vi "Get Data.vi"(8 "error in (no error)":errorcluster, 10 "Data Type":string, 11 "Communication in":refnum<class "Communication.lvclass">) -> (0 "error out":errorcluster, 3 "Communication out":refnum<class "Communication.lvclass">)   [LabVIEW 2023, in "Communication.lvclass"]
uses:
  Communication.lvclass
  Data/Data.lvclass
  Controls/User Event Operation.ctl
  Downloads/Sample PC Template/Sample PC Template/Typedefs/Data.ctl
  Communication.lvclass/Communication.ctl
  Downloads/Sample PC Template/Sample PC Template/Sample PC Template.lvlib
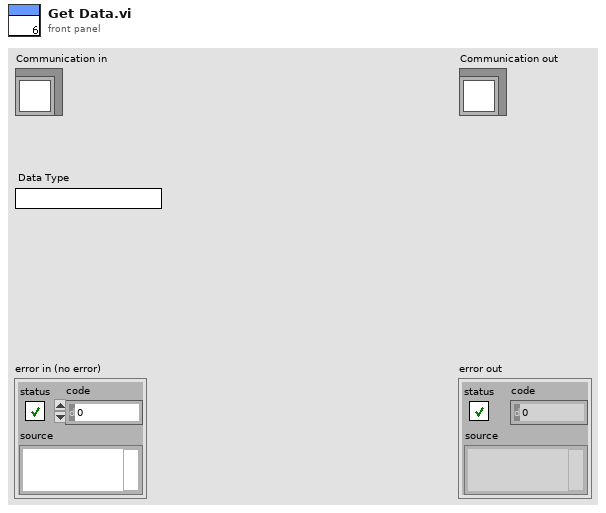
[diagram p1: front panel]
types:
  T1 = typedef "Sample PC Template.lvlib/Data.ctl" = cluster{"State":string, "Data":variant}
  T2 = typedef "User Event Operation.ctl" = enum16{"Obtain", "Generate", "Release"}
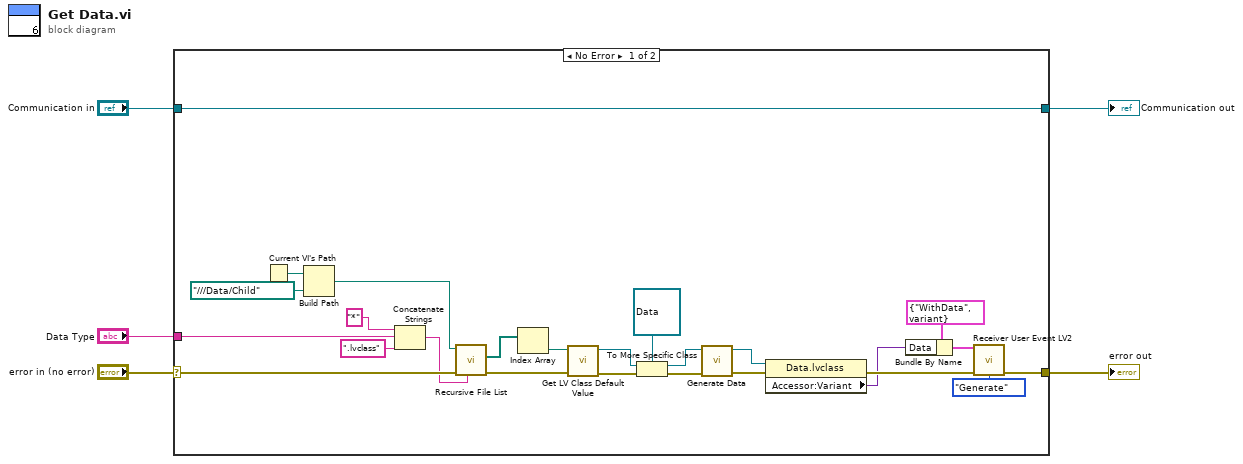
[diagram p0: block diagram]
diagram:
  n1 = case shown="No Error" "error in (no error)" {
    selector: "error in (no error)" -> [w26 w32]
    tunnel: [w16 w32] -> w4
    tunnel: [w30 w31] -> w2
    tunnel: "Communication in" -> [w30 w31]
    tunnel: "Data Type" -> [w9 _]
    frame No Error {
      n2 = Current VI's Path() -> (path=w29:path)
      n3 = Build Path(base path=w29, name or relative path=path "../../../Data/Child") -> (appended path=w11:path)
      n4 = Concatenate Strings("*" ("string"), w9, ".lvclass" ("string")) -> (w7:string)
      n5 = call <vilib>:"Recursive File List.vi"("pattern"=w7, "error in (no error)"=w26, "Folder Path"=w11) -> ("error out"=w28:errorcluster, "All Files in Dir"=w27:path[])  [unwired: 4 in, 3 out]
      n6 = Index Array(array=w27) -> (element=w6:path)  [unwired: 1 in]
      n7 = call <vilib>:"Get LV Class Default Value.vi"("error in (no error)"=w28, "class path"=w6) -> ("error out"=w24:errorcluster, "object"=w22:refnum<class>)  [unwired: 8 in]
      n8 = To More Specific Class(target class=refnum<class "Data.lvclass"> refnum ("Data.lvclass"), reference=w22, error in=w24) -> (specific class reference=w20:refnum<class "Data.lvclass">, error out=w21:errorcluster)
      n9 = call-dynamic "Generate Data.vi"("error in (no error)"=w21, "Data in"=w20) -> ("error out"=w19:errorcluster, "Data out"=w18:refnum<class "Data.lvclass">)  [unwired: 8 in]
      n10 = property class="Data.lvclass"(reference=w18, error in=w19) -> (error out=w17:errorcluster, "Accessor:Variant"=w13:variant)  [unwired: 1 out]
      n11 = Bundle By Name(cluster=T1 {"State"="WithData", "Data"=variant} ("Data"), "Data"=w13) -> (w12:T1)
      n12 = call "Receiver User Event LV2.vi"("Data"=w12, "Error In"=w17, "Operation"=User_Event_Operation."Generate") -> ("Error Out"=w16:errorcluster)  [unwired: 11 in, 1 out]
    }
    frame Error {
    }
  }
  "error out" <- w4
  "Communication out" <- w2
